vi "BLDC State to Pin.vi"(0 "Enable":refnum<k21>, 1 "Drive Pin":refnum<k21>, 2 "Compare Value":u16, 3 "State":enum16{"H", "L", "Z"}(ring)=enum."Z") -> ()   [LabVIEW 2019]
uses:
  <vilib>/rvi/eio/common/nirviEmuTemplateMethod_errors.vi
  <vilib>/eio/EIONode/EIONode.xnode
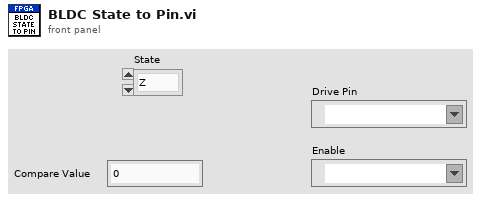
[diagram p1: front panel]
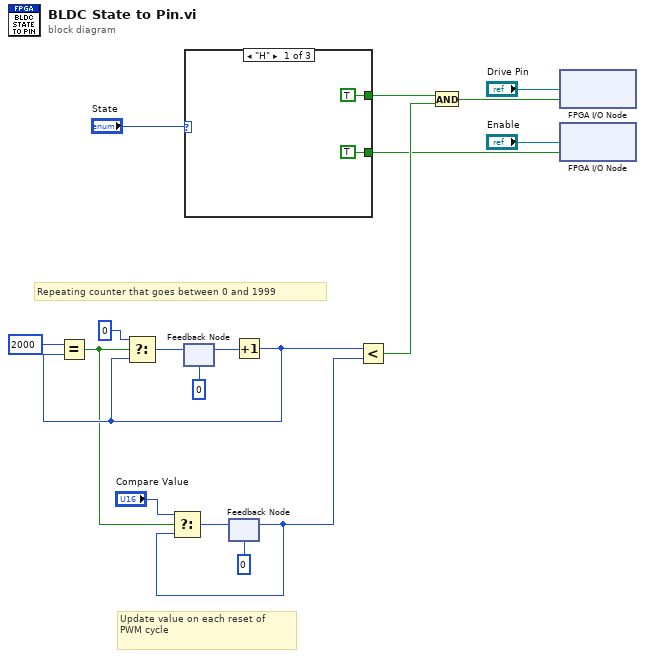
[diagram p0: block diagram]
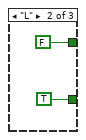
[diagram p2: hidden frame]
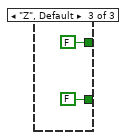
[diagram p3: hidden frame]
diagram:
  # "Repeating counter that goes between 0 and 1999"
  # "Update value on each reset of \nPWM cycle"
  n1 = feedback #1(u16 0 ("Compare Value")) -> (w10:u16)
  n2 = case shown="\"H\"" "State" {
    tunnel: [TRUE FALSE FALSE] -> w3
    tunnel: [TRUE TRUE FALSE] -> w1
    frame "H" {
    }
    frame "L" {
    }
    frame "Z", Default {
    }
  }
  n3 = feedback #2(u16 0 ("Compare Value")) -> (w6:u16)
  n4 = Increment(x=w10) -> (x+1=w7:u16)
  n5 = Equal?(x=u16 2000 ("Compare Value"), y=w7) -> (x = y?=w5:bool)
  n6 = Select(t=u16 0, s=w5, f=w7) -> (s? t:f=w12:u16)
  n7 = Select(t="Compare Value", s=w5, f=w6) -> (s? t:f=w14:u16)
  n8 = feedback-in #1(w12) -> ()
  n9 = feedback-in #2(w14) -> ()
  n10 = Less?(x=w7, y=w6) -> (x < y?=w4:bool)
  n11 = And(x=w3, y=w4) -> (x .and. y?=w2:bool)
  n12 = xnode "FPGA I/O Node"("I/O项"=w2, "FPGA I/O输入"="Drive Pin") -> ()  [unwired: 1 out]
  n13 = xnode "FPGA I/O Node"("I/O项"=w1, "FPGA I/O输入"="Enable") -> ()  [unwired: 1 out]
